vi "State Process.vi"(8 "error in (no error)":errorcluster, 11 "View Model":T1) -> (0 "error out":errorcluster, 3 "View Model":T1)   [LabVIEW 2017]
doc: "Perform actions specific to a state"
uses:
  View Model/Controls/View Model.ctl
  Error Handler/Controls/Error Model.ctl
  Error Handler/Controls/Error Type.ctl
  View Model/Controls/Shared Model.ctl
  Controls/Elevator Model.ctl
  Controls/Controller Overhead.ctl
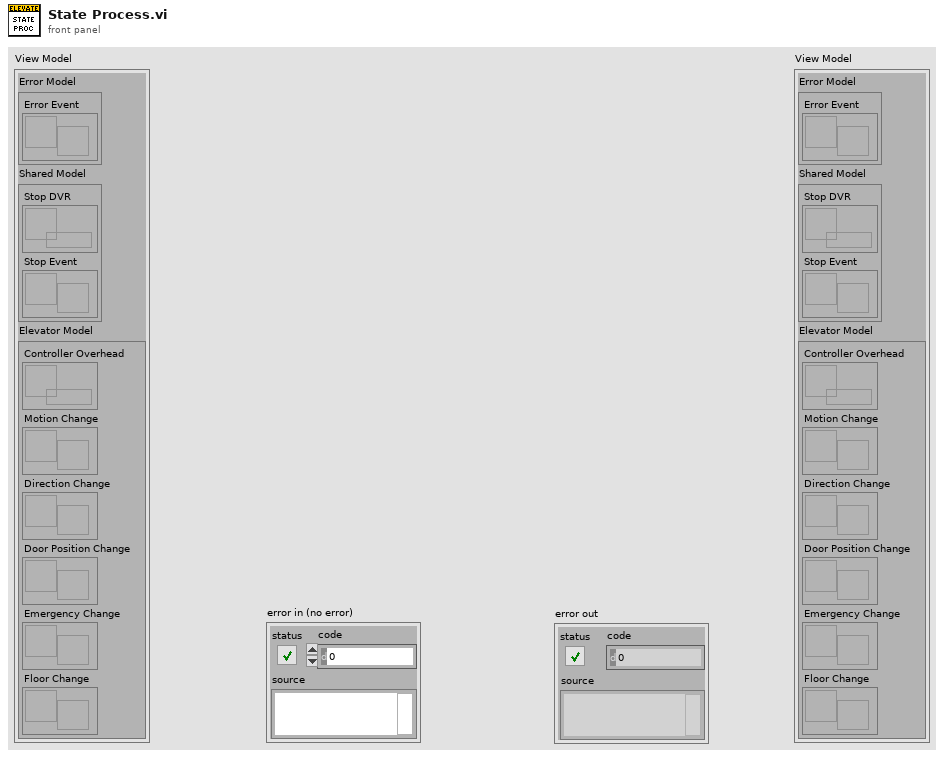
[diagram p1: front panel]
types:
  T1 = typedef "View Model.ctl" = cluster{"Error Model":T2, "Shared Model":T3, "Elevator Model":T4}
  T2 = typedef "Error Model.ctl" = cluster{"Error Event":refnum<user-event>}
  T3 = typedef "Shared Model.ctl" = cluster{"Stop DVR":refnum<data-value>, "Stop Event":refnum<user-event>}
  T4 = typedef "Elevator Model.ctl" = cluster{"Controller Overhead":refnum<data-value>, "Motion Change":refnum<user-event>, "Direction Change":refnum<user-event>, "Door Position Change":refnum<user-event>, "Emergency Change":refnum<user-event>, "Floor Change":refnum<user-event>}
  T5 = enum16{"Idle", "Open Doors", "Close Doors", "Travel", "Emergency"}
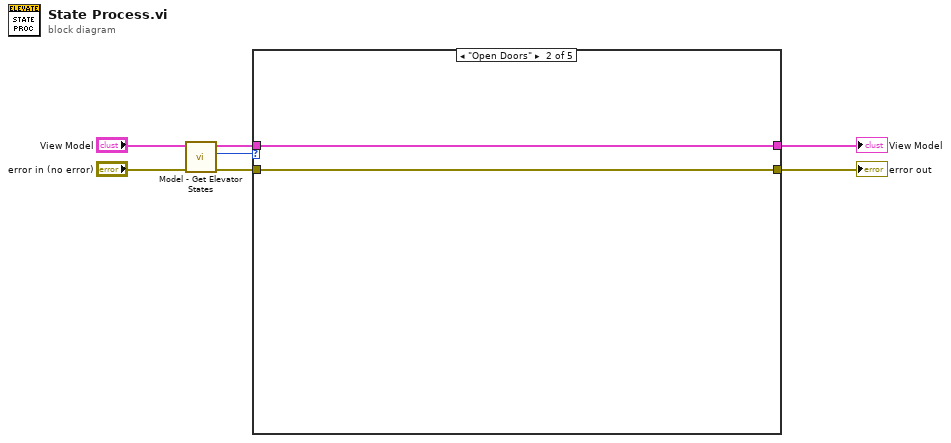
[diagram p0: block diagram]
diagram:
  n1 = call "Model - Get Elevator States.vi"("error in (no error)"="error in (no error)", "View Model"="View Model") -> ("error out"=w4:errorcluster, "Elevator State"=w6:T5, "View Model"=w5:T1)  [unwired: 6 in, 1 out]
  n2 = case shown="\"Open Doors\"" w6 {
    tunnel: w5 -> [w8 w10 w11 w12 w13]
    tunnel: w4 -> [_ w9 _ _ _]
    tunnel: [w8 w10 w11 w12 w13] -> w2
    tunnel: [_ w9 _ _ _] -> w1
    frame "Idle", Default {
    }
    frame "Open Doors" {
    }
    frame "Close Doors" {
    }
    frame "Travel" {
    }
    frame "Emergency" {
    }
  }
  "error out" <- w1
  "View Model" <- w2
